vi "Begin.vi"(11 "Image Size":T1=enum."160x120") -> (0 "error out":errorcluster)   [LabVIEW 2011]
doc: "Called before other user functions, this VI is expected to open initial I/O refnums, load in file data, and do all program initialization. Notice that the <B>error out</B> terminal is simply used for data flow. Wiring it to other structures or subVIs ensures that this VI runs first."
uses:
  <vilib>/Rock Robotics/WPI/Camera/WPI_CameraImageSize.ctl
  <vilib>/Rock Robotics/SystemInterfaces/DIO/FPGA_DIOPWMChannel.ctl
  <vilib>/Rock Robotics/SystemInterfaces/Typedef/FPGA_TypedefDigitalModule.ctl
  <vilib>/Rock Robotics/WPI/Joystick/WPI_JoystickDeviceEnum.ctl
  <vilib>/Rock Robotics/SystemInterfaces/DIO/FPGA_DIOChannel.ctl
  <vilib>/Rock Robotics/WPI/Encoder/WPI_EncoderType.ctl
  <vilib>/Rock Robotics/SystemInterfaces/AI/FPGA_AIChannel.ctl
  <vilib>/Rock Robotics/SystemInterfaces/Typedef/FPGA_TypedefAnalogModule.ctl
  <vilib>/Rock Robotics/SystemInterfaces/AI/FPGA_AIGyroChannel.ctl
  <vilib>/Rock Robotics/WPI/RobotDrive/WPI_RobotDriveOpen2MotorWithVictor.vi
  <vilib>/Rock Robotics/WPI/MotorControl/WPI_MotorControlOpen Victor.vi
  <vilib>/Rock Robotics/WPI/MotorControl/WPI_MotorControlOpen Jaguar.vi
  <vilib>/Rock Robotics/WPI/Counter/WPI_CounterDigitalInputToDigitalSource.vi
  Robot Global Data.vi
  <vilib>/Rock Robotics/WPI/Camera/WPI_CameraWhite Balance Values.ctl
  <vilib>/Rock Robotics/WPI/Camera/WPI_CameraExposure Values.ctl
  <vilib>/Rock Robotics/WPI/Camera/WPI_CameraFrameRate.ctl
panel:
  in  "Image Size 2":T1=enum."160x120"
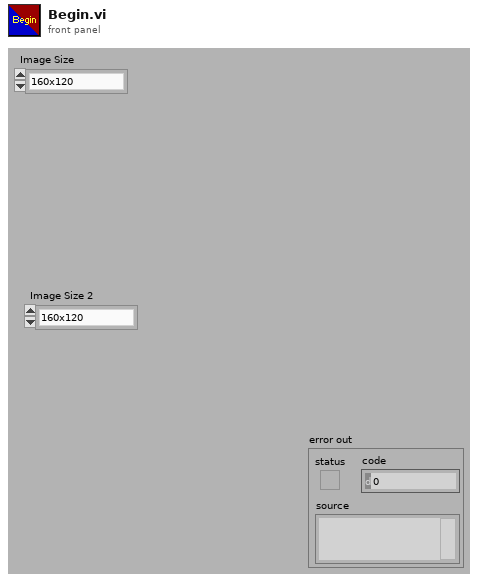
[diagram p1: front panel]
types:
  T1 = typedef "WPI_CameraImageSize.ctl" = enum16{"640x480", "320x240", "160x120"}
  T2 = typedef "FPGA_DIOChannel.ctl" = enum8{"DIO 1", "DIO 2", "DIO 3", "DIO 4", "DIO 5", "DIO 6", "DIO 7", "DIO 8", "DIO 9", "DIO 10", "DIO 11", "DIO 12", "DIO 13", "DIO 14", "Invalid"}
  T3 = typedef "FPGA_AIGyroChannel.ctl" = enum8{"AI 1", "AI 2", "Invalid"}
  T4 = typedef "WPI_EncoderType.ctl" = enum16{"1x", "2x", "4x"}
  T5 = typedef "FPGA_TypedefAnalogModule.ctl" = enum16{"Analog Module 1", "Analog Module 2"}
  T6 = typedef "FPGA_AIChannel.ctl" = enum8{"AI 1", "AI 2", "AI 3", "AI 4", "AI 5", "AI 6", "AI 7", "AI 8", "Invalid"}
  T7 = typedef "FPGA_DIOPWMChannel.ctl" = enum8{"PWM 1", "PWM 2", "PWM 3", "PWM 4", "PWM 5", "PWM 6", "PWM 7", "PWM 8", "PWM 9", "PWM 10", "Invalid"}
  T8 = typedef "WPI_JoystickDeviceEnum.ctl" = enum16{"USB 1", "USB 2", "USB 3", "USB 4", "Kinect 1", "Kinect 2"}
  T9 = typedef "FPGA_TypedefDigitalModule.ctl" = enum16{"Digital Module 1", "Digital Module 2"}
  T10 = typedef "WPI_CameraFrameRate.ctl" = u32
  T11 = typedef "WPI_CameraExposure Values.ctl" = enum16{"Auto", "Flicker-free 50 Hz", "Flicker-free 60 Hz", "Hold current"}
  T12 = typedef "WPI_CameraWhite Balance Values.ctl" = enum16{"Auto", "Fixed indoor", "Fixed outdoor 1", "Fixed outdoor 2", "Fixed fluorescent 1", "Fixed fluorescent 2", "Hold current"}
  T13 = typedef "WPI_CameraDevRef.ctl" = cluster{"Camera Address":string, "CameraStatus":errorcluster, "Acquire Image Notifier":refnum<notifier>}
  T14 = typedef "WPI_DigitalInputDevRef.ctl" = cluster{"DevStatus":errorcluster, "DIO Channel":T2, "Digital Module":T9}
  T15 = typedef "FPGA_CounterEncoderSourceConvertionLVSourceType.ctl" = cluster{"DevStatus":errorcluster, "AnalogTriggerMode?":bool, "DigitalMode":cluster{"Digital Module":T9, "DIO Channel":T16}, "AnalogTriggerMode":cluster{"AnalogTriggerIndex":T17, "OutputType":T18}}
  T16 = typedef "FPGA_DIODigitalSourceChannel.ctl" = enum8{"DIO 1", "DIO 2", "DIO 3", "DIO 4", "DIO 5", "DIO 6", "DIO 7", "DIO 8", "DIO 9", "DIO 10", "DIO 11", "DIO 12", "DIO 13", "DIO 14", "Disabled"}
  T17 = typedef "FPGA_AnalogTriggerIndex.ctl" = enum8{"Trig 0", "Trig 1", "Trig 2", "Trig 3", "Trig 4", "Trig 5", "Trig 6", "Trig 7", "Invalid"}
  T18 = typedef "FPGA_AnalogTriggerOutType.ctl" = enum16{"InWindow", "TriggerState", "Rising", "Falling"}
  T19 = typedef "WPI_JoystickDevRef.ctl" = cluster{"Device":T8}
  T20 = typedef "WPI_MotorControlDeviceRef.ctl" = cluster{"DeviceStatus":errorcluster, "Type":enum16{"PWM", "CAN"}, "PWM":cluster{"Digital Module":T9, "PWM Channel":T7, "DeadBand":T21}, "CAN":cluster{"Device Number":u8, "Control Mode":T22, "Semaphore":T23, "Max Vout":dbl}, "Invert":bool, "TransformRef":T24, "InvTransformRef":T24}
  T21 = typedef "WPI_PWMDeadband.ctl" = cluster{"Name":string, "maxPositivePwm":i32, "minPositivePwm":i32, "centerPwm":i32, "maxNegativePwm":i32, "minNegativePwm":i32, "angularRange":u16}
  T22 = typedef "WPI_CANJaguar_ControlMode.ctl" = enum8{"Percent VBus", "Current", "Speed", "Position", "Voltage"}
  T23 = typedef "Semaphore RefNum" = refnum<k1>
  T24 = typedef "WPI_PWMTransform_ConPane.ctl" = refnum<vi>
  T25 = typedef "WPI_UltrasonicDeviceRef.ctl" = cluster{"DevStatus":errorcluster, "Ping Digital Module":T9, "Echo Digital Module":T9, "Ping Channel":T2, "Echo Channel":T2, "CntIndex":T26}
  T26 = typedef "FPGA_CounterCtrSystemIndex.ctl" = enum8{"Ctr 0", "Ctr 1", "Ctr 2", "Ctr 3", "Ctr 4", "Ctr 5", "Ctr 6", "Ctr 7", "Invalid"}
  T27 = typedef "WPI_EncoderDevRef.ctl" = cluster{"DevStatus":errorcluster, "EncoderIndex":T28, "CounterIndex":T26, "DistancePerCount":dbl, "Decoding Type":T4}
  T28 = typedef "FPGA_EncoderIdx.ctl" = enum8{"Enc 0", "Enc 1", "Enc 2", "Enc 3", "Invalid"}
  T29 = typedef "WPI_RobotDriveDevRef.ctl" = cluster{"DevStatus":errorcluster, "Motors[]":T20[], "Square Inputs":bool, "Max Output":dbl, "Isochronous":bool}
  T30 = typedef "WPI_AnalogChannelDevRef.ctl" = cluster{"DevStatus":errorcluster, "Analog Module":T5, "Analog Channel":T6}
  T31 = typedef "WPI_GyroDevRef.ctl" = cluster{"DevStatus":errorcluster, "Analog Module":T5, "Analog Channel":T6, "Offset":dbl, "Gain (VoltsPerDegree/Second)":dbl}
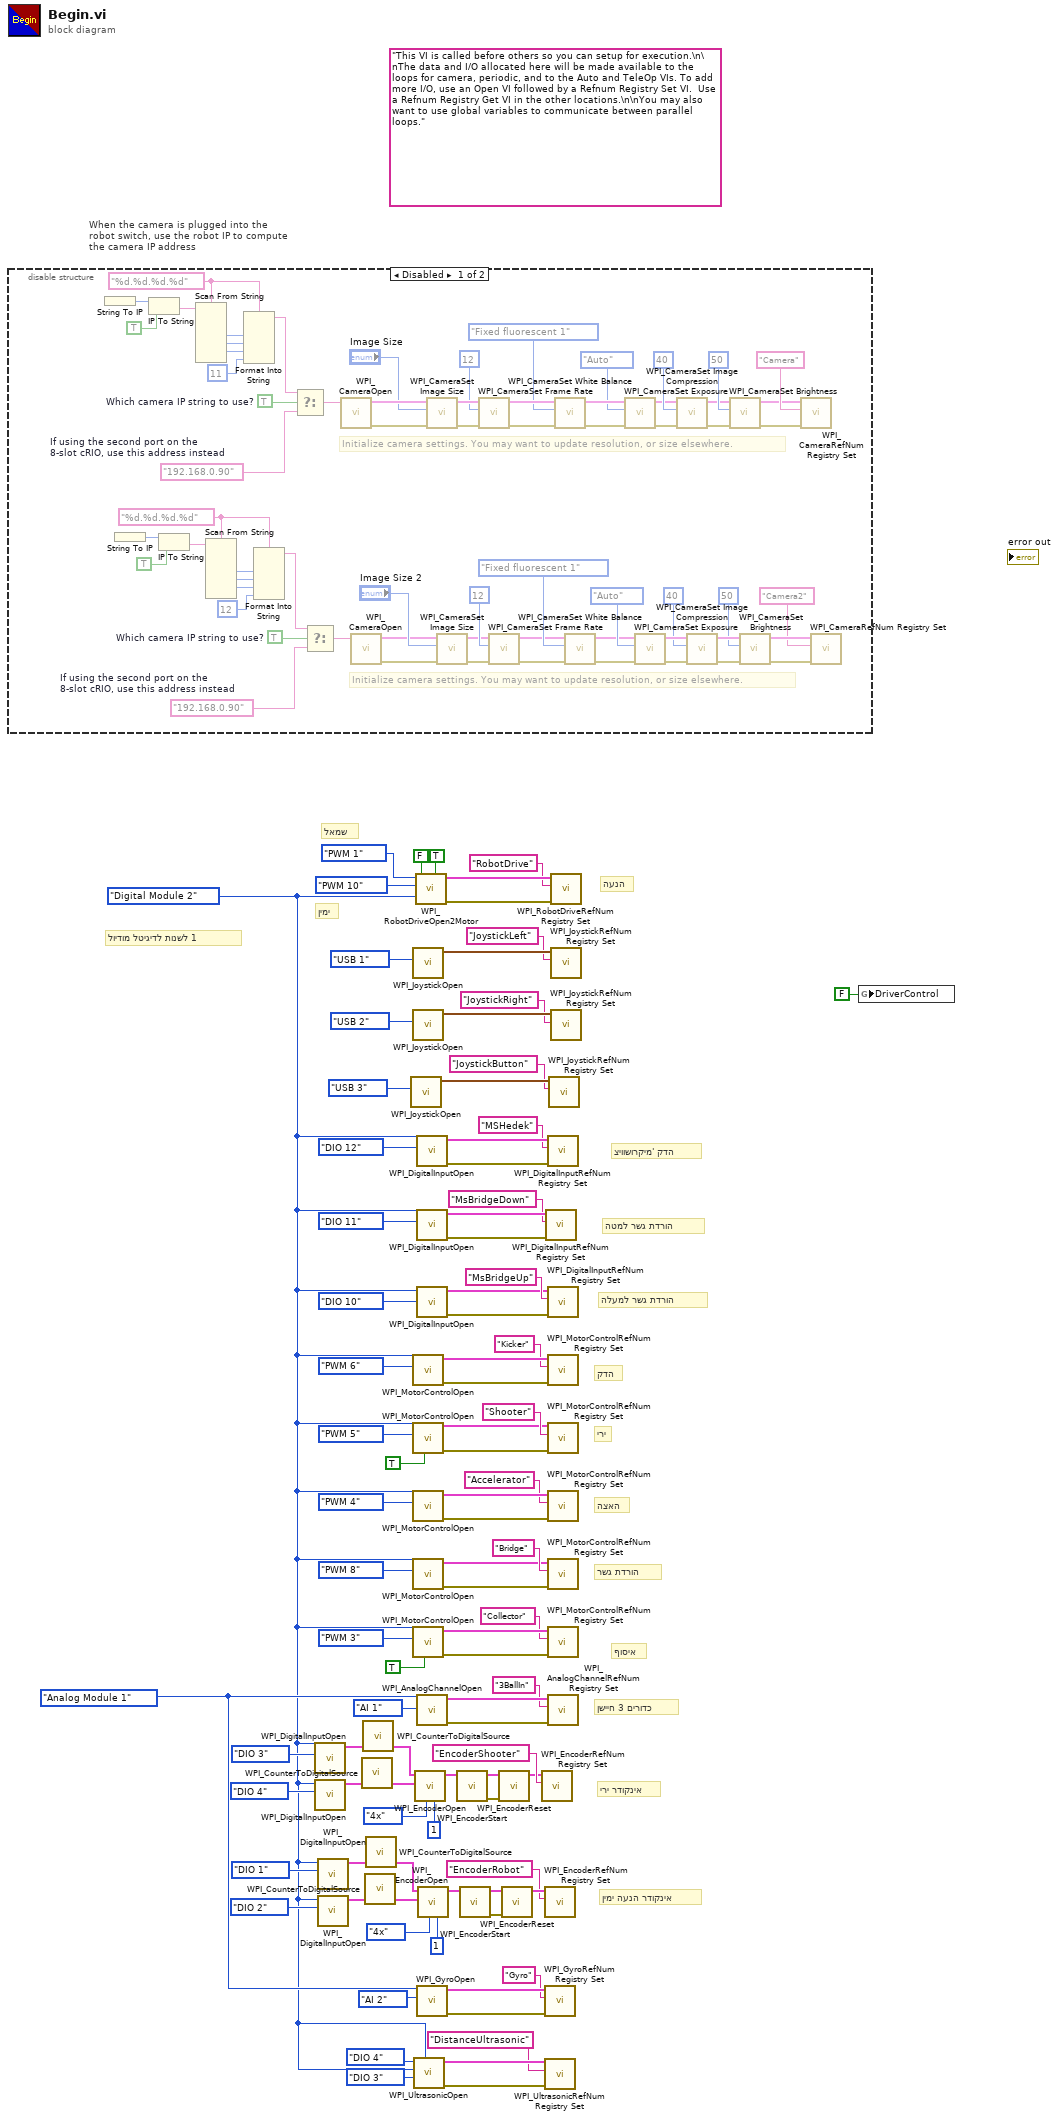
[diagram p0: block diagram]
diagram:
  w10 = FPGA_TypedefAnalogModule."Analog Module 1" ("Analog Module (Module 1)")
  w7 = FPGA_TypedefDigitalModule."Digital Module 2" ("Digital Module (Module 1)")
  (unwired) "This VI is called before others so you can setup for execution.\n\nThe data and I/O allocated here will be made available to the loops for camera, periodic, and to the Auto and TeleOp VIs. To add more I/O, use an Open VI followed by a Refnum Registry Set VI.  Use a Refnum Registry Get VI in the other locations.\n\nYou may also want to use global variables to communicate between parallel loops."
  # "אינקודר הנעה ימין"
  # "איסוף"
  # "When the camera is plugged into the\nrobot switch, use the robot IP to compute\nthe camera IP address"
  # "לשנות לדיגיטל מודיול 1"
  # "אינקודר ירי"
  # "מיקרושוויצ' הדק"
  # "הורדת גשר למטה"
  # "הורדת גשר למעלה"
  # "ימין"
  # "שמאל"
  # "הנעה"
  # "חיישן 3 כדורים"
  # "הורדת גשר"
  # "האצה"
  # "ירי"
  # "הדק"
  n1 = disable-structure shown="Disabled" {
    frame Disabled {
      w125 = TRUE  # Which camera IP string to use?
      w121 = "%d.%d.%d.%d" ("format string")
      w124 = "192.168.0.90"  # If using the second port on the 8-slot cRIO, use this address instead
      w126 = TRUE  # Which camera IP string to use?
      w130 = "%d.%d.%d.%d" ("format string")
      w127 = "192.168.0.90"  # If using the second port on the 8-slot cRIO, use this address instead
      # "Initialize camera settings. You may want to update resolution, or size elsewhere."
      # "Initialize camera settings. You may want to update resolution, or size elsewhere."
      n2 = String To IP() -> (0:w137:u32)  [unwired: 1 in]
      n3 = String To IP() -> (0:w114:u32)  [unwired: 1 in]
      n4 = IP To String(1:TRUE ("dot notation? (F)"), 2:w137) -> (0:w135:string)
      n5 = IP To String(1:TRUE ("dot notation? (F)"), 2:w114) -> (0:w116:string)
      n6 = Scan From String(format string=w130, input string=w135) -> (output 1=w134:i32, output 2=w133:i32, output 3=w132:i32)  [unwired: 7 in, 3 out]
      n7 = Scan From String(format string=w121, input string=w116) -> (output 1=w117:i32, output 2=w118:i32, output 3=w119:i32)  [unwired: 7 in, 3 out]
      n8 = Format Into String(format string=w130, w134, w133, w132, 11 ("Compression")) -> (resulting string=w128:string)  [unwired: 2 in, 1 out]
      n9 = Format Into String(format string=w121, w117, w118, w119, 12 ("Compression")) -> (resulting string=w123:string)  [unwired: 2 in, 1 out]
      n10 = Select(t=w128, s=w126, f=w127) -> (s? t:f=w129:string)
      n11 = Select(t=w123, s=w125, f=w124) -> (s? t:f=w122:string)
      n12 = call <vilib>:"WPI_CameraOpen.vi"("Camera Address"=w129) -> ("error out"=w149:errorcluster, "CameraDevRef"=w150:T13)  [unwired: 1 in, 8 out]
      n13 = call <vilib>:"WPI_CameraOpen.vi"("Camera Address"=w122) -> ("error out"=w102:errorcluster, "CameraDevRef"=w101:T13)  [unwired: 1 in, 8 out]
      n14 = call <vilib>:"WPI_CameraSet Image Size.vi"("error in (no error)"=w149, "Image Size"="Image Size", "CameraDevRef"=w150) -> ("error out"=w148:errorcluster, "CameraDevRef Out"=w151:T13)  [unwired: 7 out]
      n15 = call <vilib>:"WPI_CameraSet Image Size.vi"("error in (no error)"=w102, "Image Size"="Image Size 2", "CameraDevRef"=w101) -> ("error out"=w103:errorcluster, "CameraDevRef Out"=w100:T13)  [unwired: 7 out]
      n16 = call <vilib>:"WPI_CameraSet Frame Rate.vi"("error in (no error)"=w148, "Frame Rate (fps)"=T10 12, "CameraDevRef"=w151) -> ("error out"=w147:errorcluster, "CameraDevRef Out"=w153:T13)  [unwired: 7 out]
      n17 = call <vilib>:"WPI_CameraSet Frame Rate.vi"("error in (no error)"=w103, "Frame Rate (fps)"=T10 12, "CameraDevRef"=w100) -> ("error out"=w104:errorcluster, "CameraDevRef Out"=w98:T13)  [unwired: 7 out]
      n18 = call <vilib>:"WPI_CameraSet White Balance.vi"("error in (no error)"=w147, "White Balance"=WPI_CameraWhite_Balance_Values."Fixed fluorescent 1", "CameraDevRef"=w153) -> ("error out"=w146:errorcluster, "CameraDevRef Out"=w152:T13)  [unwired: 7 out]
      n19 = call <vilib>:"WPI_CameraSet White Balance.vi"("error in (no error)"=w104, "White Balance"=WPI_CameraWhite_Balance_Values."Fixed fluorescent 1", "CameraDevRef"=w98) -> ("error out"=w105:errorcluster, "CameraDevRef Out"=w99:T13)  [unwired: 7 out]
      n20 = call <vilib>:"WPI_CameraSet Exposure.vi"("error in (no error)"=w146, "Exposure"=WPI_CameraExposure_Values."Auto", "CameraDevRef"=w152) -> ("error out"=w145:errorcluster, "CameraDevRef Out"=w155:T13)  [unwired: 7 out]
      n21 = call <vilib>:"WPI_CameraSet Exposure.vi"("error in (no error)"=w105, "Exposure"=WPI_CameraExposure_Values."Auto", "CameraDevRef"=w99) -> ("error out"=w106:errorcluster, "CameraDevRef Out"=w96:T13)  [unwired: 7 out]
      n22 = call <vilib>:"WPI_CameraSet Image Compression.vi"("error in (no error)"=w145, "Compression"=40, "CameraDevRef"=w155) -> ("error out"=w144:errorcluster, "CameraDevRef Out"=w154:T13)  [unwired: 7 out]
      n23 = call <vilib>:"WPI_CameraSet Image Compression.vi"("error in (no error)"=w106, "Compression"=40, "CameraDevRef"=w96) -> ("error out"=w107:errorcluster, "CameraDevRef Out"=w97:T13)  [unwired: 7 out]
      n24 = call <vilib>:"WPI_CameraSet Brightness.vi"("error in (no error)"=w144, "Brightness"=50, "CameraDevRef"=w154) -> ("error out"=w142:errorcluster, "CameraDevRef Out"=w143:T13)  [unwired: 7 out]
      n25 = call <vilib>:"WPI_CameraSet Brightness.vi"("error in (no error)"=w107, "Brightness"=50, "CameraDevRef"=w97) -> ("error out"=w109:errorcluster, "CameraDevRef Out"=w108:T13)  [unwired: 7 out]
      n26 = call <vilib>:"WPI_CameraRefNum Registry Set.vi"("error in (no error)"=w142, "refnum name"="Camera", "CameraDevRef"=w143) -> ()  [unwired: 9 out]
      n27 = call <vilib>:"WPI_CameraRefNum Registry Set.vi"("error in (no error)"=w109, "refnum name"="Camera2", "CameraDevRef"=w108) -> ()  [unwired: 9 out]
    }
    frame Enabled {
    }
  }
  n28 = call <vilib>:"WPI_DigitalInputOpen.vi"("DIO Channel"=FPGA_DIOChannel."DIO 3", "Digital Module (Module 1)"=w7) -> ("DigitalInputDevRef"=w52:T14)  [unwired: 8 in, 1 out]
  n29 = call <vilib>:"WPI_DigitalInputOpen.vi"("DIO Channel"=FPGA_DIOChannel."DIO 4", "Digital Module (Module 1)"=w7) -> ("DigitalInputDevRef"=w50:T14)  [unwired: 8 in, 1 out]
  n30 = call <vilib>:"WPI_DigitalInputOpen.vi"("DIO Channel"=FPGA_DIOChannel."DIO 1", "Digital Module (Module 1)"=w7) -> ("DigitalInputDevRef"=w15:T14)  [unwired: 8 in, 1 out]
  n31 = call <vilib>:"WPI_DigitalInputOpen.vi"("DIO Channel"=FPGA_DIOChannel."DIO 2", "Digital Module (Module 1)"=w7) -> ("DigitalInputDevRef"=w17:T14)  [unwired: 8 in, 1 out]
  n32 = call-poly <vilib>:"WPI_CounterToDigitalSource.vi"("DigitalInputDevRef"=w50) -> ("Digital Source"=w49:T15)  [unwired: 6 in]
  n33 = call-poly <vilib>:"WPI_CounterToDigitalSource.vi"("DigitalInputDevRef"=w52) -> ("Digital Source"=w51:T15)  [unwired: 6 in]
  n34 = call-poly <vilib>:"WPI_CounterToDigitalSource.vi"("DigitalInputDevRef"=w17) -> ("Digital Source"=w18:T15)  [unwired: 6 in]
  n35 = call-poly <vilib>:"WPI_CounterToDigitalSource.vi"("DigitalInputDevRef"=w15) -> ("Digital Source"=w16:T15)  [unwired: 6 in]
  n36 = call <vilib>:"WPI_JoystickOpen.vi"("JoystickDevice"=WPI_JoystickDeviceEnum."USB 3") -> ("JoystickDevRef"=w81:T19)  [unwired: 10 in]
  n37 = call <vilib>:"WPI_JoystickOpen.vi"("JoystickDevice"=WPI_JoystickDeviceEnum."USB 1") -> ("JoystickDevRef"=w85:T19)  [unwired: 10 in]
  n38 = call <vilib>:"WPI_JoystickOpen.vi"("JoystickDevice"=WPI_JoystickDeviceEnum."USB 2") -> ("JoystickDevRef"=w82:T19)  [unwired: 10 in]
  n39 = call-poly <vilib>:"WPI_MotorControlOpen.vi"("PWM Channel"=FPGA_DIOPWMChannel."PWM 6", "Digital Module (Module 1)"=w7) -> ("error out"=w76:errorcluster, "MotorControlDeviceRef"=w75:T20)  [unwired: 8 in]
  n40 = call-poly <vilib>:"WPI_MotorControlOpen.vi"("Invert"=TRUE, "PWM Channel"=FPGA_DIOPWMChannel."PWM 5", "Digital Module (Module 1)"=w7) -> ("error out"=w69:errorcluster, "MotorControlDeviceRef"=w70:T20)  [unwired: 7 in]
  n41 = call-poly <vilib>:"WPI_MotorControlOpen.vi"("PWM Channel"=FPGA_DIOPWMChannel."PWM 4", "Digital Module (Module 1)"=w7) -> ("error out"=w68:errorcluster, "MotorControlDeviceRef"=w67:T20)  [unwired: 8 in]
  n42 = call-poly <vilib>:"WPI_MotorControlOpen.vi"("PWM Channel"=FPGA_DIOPWMChannel."PWM 8", "Digital Module (Module 1)"=w7) -> ("error out"=w61:errorcluster, "MotorControlDeviceRef"=w62:T20)  [unwired: 8 in]
  n43 = call-poly <vilib>:"WPI_MotorControlOpen.vi"("Invert"=TRUE, "PWM Channel"=FPGA_DIOPWMChannel."PWM 3", "Digital Module (Module 1)"=w7) -> ("error out"=w60:errorcluster, "MotorControlDeviceRef"=w59:T20)  [unwired: 7 in]
  n44 = call <vilib>:"WPI_UltrasonicOpen.vi"("Ping Digital Module (Module 1)"=w7, "Echo DIO Channel"=FPGA_DIOChannel."DIO 3", "Echo Digital Module (Module 1)"=w7, "Ping DIO Channel"=FPGA_DIOChannel."DIO 4") -> ("error out"=w9:errorcluster, "UltrasonicDevRef"=w8:T25)  [unwired: 6 in]
  n45 = call <vilib>:"WPI_EncoderOpen.vi"("DistancePerCount"=1, "Decoding Type"=WPI_EncoderType."4x", "BSource"=w49, "ASource"=w51) -> ("EncoderDevRef"=w32:T27)  [unwired: 6 in, 1 out]
  n46 = call-poly <vilib>:"WPI_RobotDriveOpen2Motor.vi"("Right Motor Inverted"=TRUE, "Left Motor Inverted"=FALSE, "Digital Module (Module 1)"=w7, "Right Motor"=FPGA_DIOPWMChannel."PWM 10", "Left Motor"=FPGA_DIOPWMChannel."PWM 1") -> ("error out"=w92:errorcluster, "RobotDriveDevRef"=w91:T29)  [unwired: 5 in]
  n47 = call <vilib>:"WPI_DigitalInputOpen.vi"("DIO Channel"=FPGA_DIOChannel."DIO 12", "Digital Module (Module 1)"=w7) -> ("error out"=w56:errorcluster, "DigitalInputDevRef"=w55:T14)  [unwired: 8 in]
  n48 = call <vilib>:"WPI_DigitalInputOpen.vi"("DIO Channel"=FPGA_DIOChannel."DIO 11", "Digital Module (Module 1)"=w7) -> ("error out"=w37:errorcluster, "DigitalInputDevRef"=w36:T14)  [unwired: 8 in]
  n49 = call <vilib>:"WPI_DigitalInputOpen.vi"("DIO Channel"=FPGA_DIOChannel."DIO 10", "Digital Module (Module 1)"=w7) -> ("error out"=w38:errorcluster, "DigitalInputDevRef"=w39:T14)  [unwired: 8 in]
  n50 = call <vilib>:"WPI_AnalogChannelOpen.vi"("Analog Channel"=FPGA_AIChannel."AI 1", "Analog Module (Module 1)"=w10) -> ("error out"=w45:errorcluster, "AIDeviceRef"=w44:T30)  [unwired: 8 in]
  n51 = call <vilib>:"WPI_GyroOpen.vi"("Analog Channel"=FPGA_AIGyroChannel."AI 2", "Analog Module (Module 1)"=w10) -> ("error out"=w14:errorcluster, "GyroDevRef"=w13:T31)  [unwired: 7 in, 1 out]
  n52 = call <vilib>:"WPI_EncoderOpen.vi"("DistancePerCount"=1, "Decoding Type"=WPI_EncoderType."4x", "BSource"=w18, "ASource"=w16) -> ("EncoderDevRef"=w23:T27)  [unwired: 6 in, 1 out]
  n53 = call <vilib>:"WPI_EncoderStart.vi"("EncoderDevRef"=w32) -> ("error out"=w31:errorcluster, "EncoderDevRef"=w30:T27)  [unwired: 9 in]
  n54 = call <vilib>:"WPI_EncoderStart.vi"("EncoderDevRef"=w23) -> ("error out"=w24:errorcluster, "EncoderDevRef"=w25:T27)  [unwired: 9 in]
  n55 = call <vilib>:"WPI_EncoderReset.vi"("error in (no error)"=w31, "EncoderDevRef"=w30) -> ("EncoderDevRef"=w29:T27)  [unwired: 8 in, 1 out]
  n56 = call <vilib>:"WPI_EncoderReset.vi"("error in (no error)"=w24, "EncoderDevRef"=w25) -> ("EncoderDevRef"=w26:T27)  [unwired: 8 in, 1 out]
  n57 = call <vilib>:"WPI_EncoderRefNum Registry Set.vi"("refnum name"="EncoderShooter", "EncoderDevRef"=w29) -> ()  [unwired: 8 in, 2 out]
  n58 = call <vilib>:"WPI_EncoderRefNum Registry Set.vi"("refnum name"="EncoderRobot", "EncoderDevRef"=w26) -> ()  [unwired: 8 in, 2 out]
  n59 = call <vilib>:"WPI_GyroRefNum Registry Set.vi"("error in (no error)"=w14, "refnum name"="Gyro", "GyroDevRef"=w13) -> ()  [unwired: 7 in, 2 out]
  n60 = call <vilib>:"WPI_UltrasonicRefNum Registry Set.vi"("error in (no error)"=w9, "refnum name"="DistanceUltrasonic", "UltrasonicDevRef"=w8) -> ()  [unwired: 7 in, 2 out]
  n61 = call <vilib>:"WPI_DigitalInputRefNum Registry Set.vi"("error in (no error)"=w37, "refnum name"="MsBridgeDown", "DigitalInputDevRef"=w36) -> ()  [unwired: 7 in, 2 out]
  n62 = call <vilib>:"WPI_DigitalInputRefNum Registry Set.vi"("error in (no error)"=w56, "refnum name"="MSHedek", "DigitalInputDevRef"=w55) -> ()  [unwired: 7 in, 2 out]
  n63 = call <vilib>:"WPI_DigitalInputRefNum Registry Set.vi"("error in (no error)"=w38, "refnum name"="MsBridgeUp", "DigitalInputDevRef"=w39) -> ()  [unwired: 7 in, 2 out]
  n64 = call <vilib>:"WPI_MotorControlRefNum Registry Set.vi"("error in (no error)"=w76, "refnum name"="Kicker", "MotorControlDevRef"=w75) -> ()  [unwired: 7 in, 2 out]
  n65 = call <vilib>:"WPI_MotorControlRefNum Registry Set.vi"("error in (no error)"=w69, "refnum name"="Shooter", "MotorControlDevRef"=w70) -> ()  [unwired: 7 in, 2 out]
  n66 = call <vilib>:"WPI_MotorControlRefNum Registry Set.vi"("error in (no error)"=w68, "refnum name"="Accelerator", "MotorControlDevRef"=w67) -> ()  [unwired: 7 in, 2 out]
  n67 = call <vilib>:"WPI_MotorControlRefNum Registry Set.vi"("error in (no error)"=w61, "refnum name"="Bridge", "MotorControlDevRef"=w62) -> ()  [unwired: 7 in, 2 out]
  n68 = call <vilib>:"WPI_MotorControlRefNum Registry Set.vi"("error in (no error)"=w60, "refnum name"="Collector", "MotorControlDevRef"=w59) -> ()  [unwired: 7 in, 2 out]
  n69 = call <vilib>:"WPI_AnalogChannelRefNum Registry Set.vi"("error in (no error)"=w45, "refnum name"="3BallIn", "AIDeviceRef"=w44) -> ()  [unwired: 7 in, 2 out]
  n70 = call <vilib>:"WPI_JoystickRefNum Registry Set.vi"("refnum name"="JoystickButton", "JoystickDevRef"=w81) -> ()  [unwired: 8 in, 2 out]
  n71 = call <vilib>:"WPI_RobotDriveRefNum Registry Set.vi"("error in (no error)"=w92, "refnum name"="RobotDrive", "RobotDriveDevRef"=w91) -> ()  [unwired: 7 in, 2 out]
  n72 = call <vilib>:"WPI_JoystickRefNum Registry Set.vi"("refnum name"="JoystickLeft", "JoystickDevRef"=w85) -> ()  [unwired: 8 in, 2 out]
  n73 = call <vilib>:"WPI_JoystickRefNum Registry Set.vi"("refnum name"="JoystickRight", "JoystickDevRef"=w82) -> ()  [unwired: 8 in, 2 out]
  n74 = global write "Robot Global Data.vi" "DriverControl"(FALSE ("DriverControl")) -> ()
